vi "IncrementOpCount.vi"(11 "StreamData in":refnum<class "StreamData.lvclass">) -> (3 "StreamData out":refnum<class "StreamData.lvclass">)   [LabVIEW 2017, in "Stream-t'WPI_EncoderType.ctl'.lvlib" / "StreamData.lvclass"]
uses:
  <extravilib>/ChannelInstances/Stream-t'WPI_EncoderType.ctl'/StreamData.lvclass
  <extravilib>/ChannelInstances/Stream-t'WPI_EncoderType.ctl'/StreamData.lvclass/StreamData.ctl
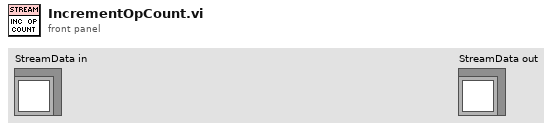
[diagram p1: front panel]
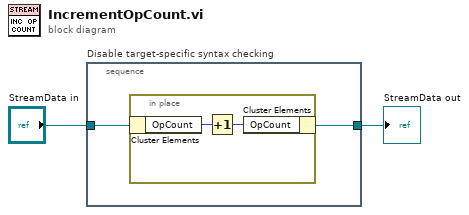
[diagram p0: block diagram]
diagram:
  n1 = stacked-sequence "Disable target-specific syntax checking" {
    tunnel: "StreamData in" -> [w4]
    tunnel: [w3] -> w1
    frame #0 {
      n2 = in-place {
        n3 = in-place-cluster #1(w4) -> ("OpCount"=w6:u32)
        n4 = Increment(x=w6) -> (x+1=w5:u32)
        n5 = in-place-cluster #1("OpCount"=w5) -> (w3:refnum<class "StreamData.lvclass">)
      }
    }
  }
  "StreamData out" <- w1
